vi "uTransport_IsValid.vi"(8 "error in (no error)":errorcluster, 11 "uTransport_Queue in":refnum<class "uTransport_Queue.lvclass">) -> (0 "error out":errorcluster, 2 "IsValid?":bool, 3 "uTransport_Queue out":refnum<class "uTransport_Queue.lvclass">)   [LabVIEW 2023, in "uLib.lvlib" / "uTransport_Queue.lvclass"]
uses:
  uTransport_Queue.lvclass
  uTransport_Queue.lvclass/uTransport_Queue.ctl
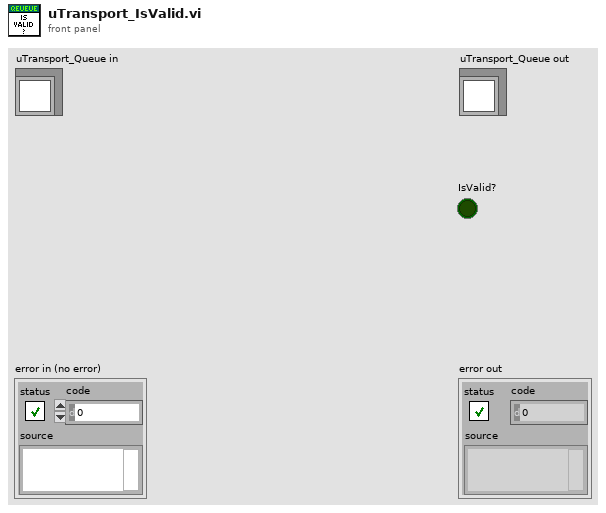
[diagram p1: front panel]
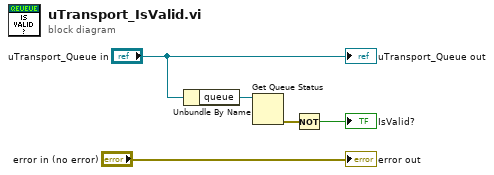
[diagram p0: block diagram]
diagram:
  n1 = Unbundle By Name("uTransport_Queue in") -> ("queue"=w1:refnum<queue>)
  n2 = Get Queue Status(queue=w1) -> (error out=w5:errorcluster)  [unwired: 2 in, 7 out]
  n3 = Not(x=w5) -> (.not. x?=→"IsValid?":bool)
  "error out" <- "error in (no error)"
  "uTransport_Queue out" <- "uTransport_Queue in"
